vi "Read Original Error Cluster.vi"(8 "error in (no error)":errorcluster, 11 "Exception Classic Error in":refnum<class "Exception Classic Error.lvclass">) -> (0 "error out":errorcluster, 2 "Original Error Cluster":errorcluster, 3 "Exception Classic Error out":refnum<class "Exception Classic Error.lvclass">)   [LabVIEW 2015, in "LV Exceptions v1.lvlib" / "Exception Classic Error.lvclass"]
uses:
  Exception Classic Error.lvclass
  Exception Classic Error.lvclass/Exception Classic Error.ctl
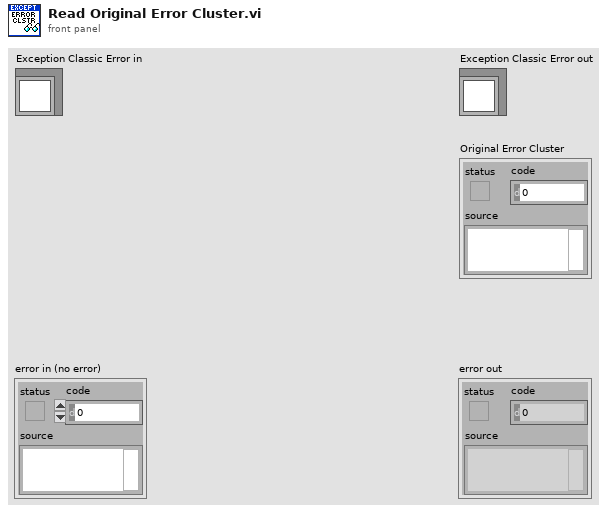
[diagram p1: front panel]
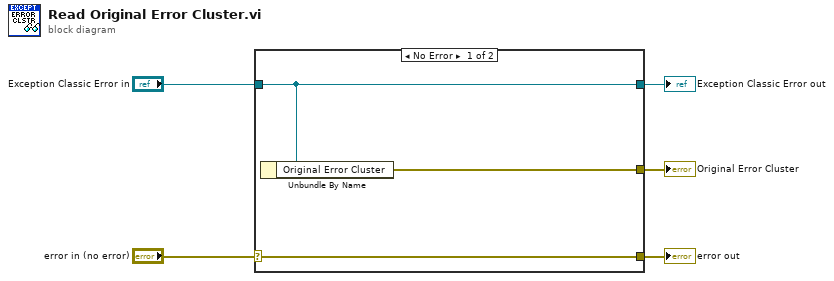
[diagram p0: block diagram]
diagram:
  n1 = case shown="No Error" "error in (no error)" {
    selector: "error in (no error)" -> [w8 w9]
    tunnel: [w8 w9] -> w4
    tunnel: [w7 w10] -> w2
    tunnel: "Exception Classic Error in" -> [w7 w10]
    tunnel: [w6 _] -> w1
    frame No Error {
      n2 = Unbundle By Name(w7) -> ("Original Error Cluster"=w6:errorcluster)
    }
    frame Error {
    }
  }
  "error out" <- w4
  "Exception Classic Error out" <- w2
  "Original Error Cluster" <- w1
